vi "Free Move.vi"(8 "Error In":errorcluster, 10 "Directions":T1, 11 "Address / Port in":i16=1 min=1 max=31 step=1) -> (0 "Error Out":errorcluster, 3 "Address / Port out":i16)   [LabVIEW 2014]
doc: "Move the motors depending on the arrow buttons pushed. BETA VERSION!!!!!"
uses:
  ESP Typedef/Direction.ctl
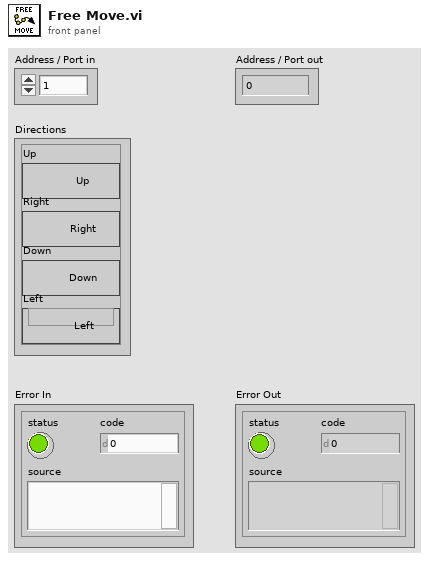
[diagram p1: front panel]
types:
  T1 = typedef "Direction.ctl" = cluster{"Up":bool, "Right":bool, "Down":bool, "Left":bool}
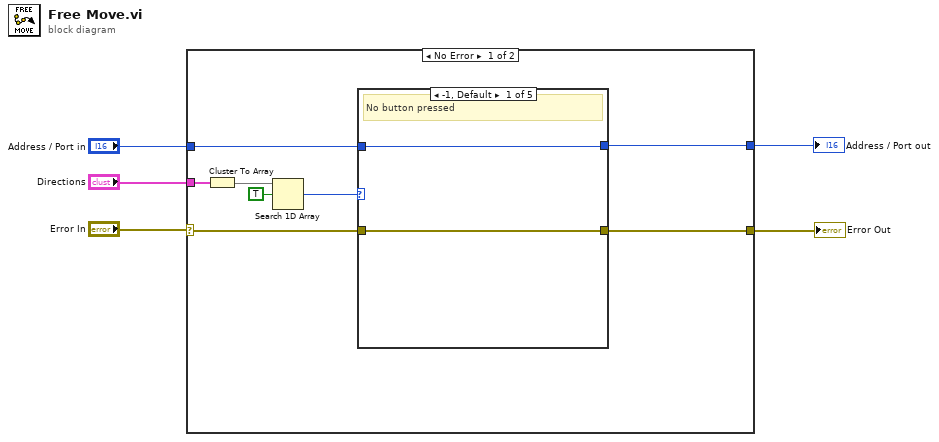
[diagram p0: block diagram]
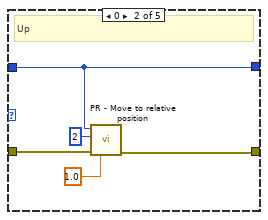
[diagram p2: hidden frame]
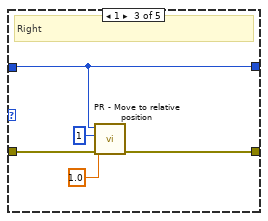
[diagram p3: hidden frame]
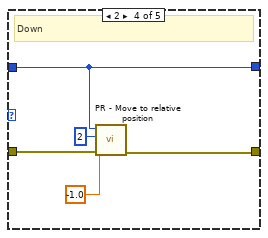
[diagram p4: hidden frame]
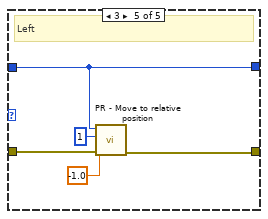
[diagram p5: hidden frame]
diagram:
  n1 = case shown="No Error" "Error In" {
    selector: "Error In" -> [w9 w37]
    tunnel: "Directions" -> [w10 _]
    tunnel: [w7 w37] -> w3
    tunnel: "Address / Port in" -> [w8 w36]
    tunnel: [w6 w36] -> w1
    frame No Error {
      n2 = Cluster To Array(cluster=w10) -> (array=w13:bool[])
      n3 = Search 1D Array(1D array=w13, element=TRUE) -> (index of element=w11:i32)  [unwired: 1 in]
      n4 = case shown="-1, Default" w11 {
        tunnel: w9 -> [w15 w20 w24 w29 w34]
        tunnel: w8 -> [w14 w17 w22 w27 w32]
        tunnel: [w15 w16 w21 w26 w31] -> w7
        tunnel: [w14 w17 w22 w27 w32] -> w6
        frame -1, Default {
          # "No button pressed"
        }
        frame 0 {
          # "Up"
          n5 = call "PR - Move to relative position.vi"("error in"=w20, "Nstep"=1.0, "Axis  #"=i8 2, "Address / Port"=w17) -> ("error out"=w16:errorcluster)  [unwired: 3 in, 2 out]
        }
        frame 1 {
          # "Right"
          n6 = call "PR - Move to relative position.vi"("error in"=w24, "Nstep"=1.0, "Axis  #"=i8 1, "Address / Port"=w22) -> ("error out"=w21:errorcluster)  [unwired: 3 in, 2 out]
        }
        frame 2 {
          # "Down"
          n7 = call "PR - Move to relative position.vi"("error in"=w29, "Nstep"=-1.0, "Axis  #"=i8 2, "Address / Port"=w27) -> ("error out"=w26:errorcluster)  [unwired: 3 in, 2 out]
        }
        frame 3 {
          # "Left"
          n8 = call "PR - Move to relative position.vi"("error in"=w34, "Nstep"=-1.0, "Axis  #"=i8 1, "Address / Port"=w32) -> ("error out"=w31:errorcluster)  [unwired: 3 in, 2 out]
        }
      }
    }
    frame Error {
    }
  }
  "Error Out" <- w3
  "Address / Port out" <- w1
